vi "Measurement.vi"(8 "error in (no error)":errorcluster, 11 "YP03-60_X in":refnum<class "YP03-60_X.lvclass">) -> (0 "error out":errorcluster, 2 "Output":dbl[](array[numeric]), 3 "YP03-60_X out":refnum<class "YP03-60_X.lvclass">)   [LabVIEW 2020, in "PowerControl.lvlib" / "YP03-60_X.lvclass"]
uses:
  YP03-60_X.lvclass
  VirtualPower/VirtualPower.lvclass
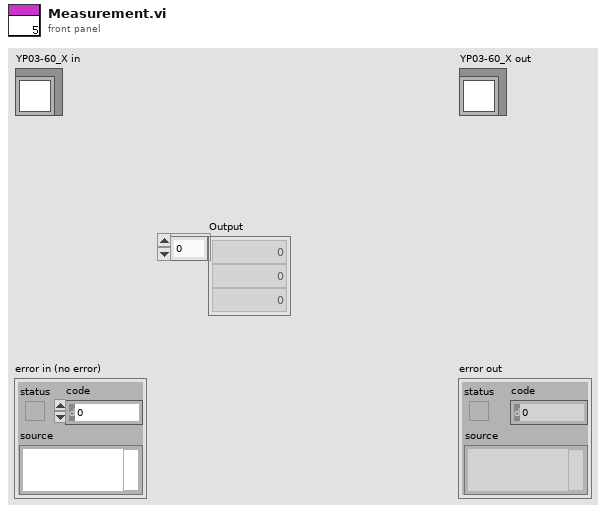
[diagram p1: front panel]
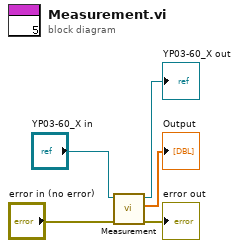
[diagram p0: block diagram]
diagram:
  n1 = call-parent "Measurement.vi"("error in (no error)"="error in (no error)", "VirtualPower in"="YP03-60_X in") -> ("error out"=→"error out":errorcluster, "Output"=→"Output":dbl[], "VirtualPower out"=→"YP03-60_X out":refnum<class "YP03-60_X.lvclass">)  [unwired: 7 in]
